vi "Configure Input Wavelength.vi"(0 "VISA resource name":refnum<visa-resource-name>, 1 "Wavelength Unit (0:NM)":u16(ring) items=["NM", "M"], 5 "Platform Slot Number (10)":i16=10 min=-1 max=255, 7 "Wavelength (0:MINimum)":i32(ring) items=["MINimum", "MAXimum", "DEFault", "User Defined Value"], 9 "User Defined Wavelength Value (1310)":dbl=1310.0, 11 "error in (no error)":errorcluster) -> (4 "VISA resource name out":refnum<visa-resource-name>, 15 "error out":errorcluster)   [LabVIEW 2018, in "LTB-1.lvlib" / "3150.lvlib"]
doc: "Configures the specific Input wavelength in meters or nanometers"
uses:
  3150.lvlib
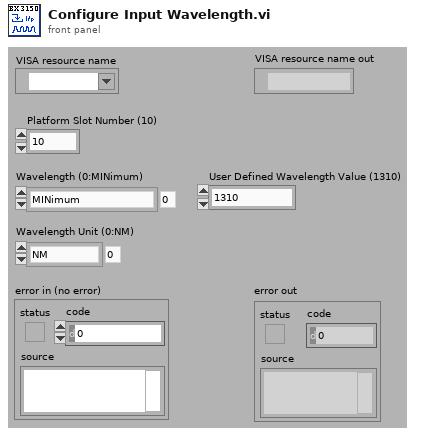
[diagram p1: front panel]
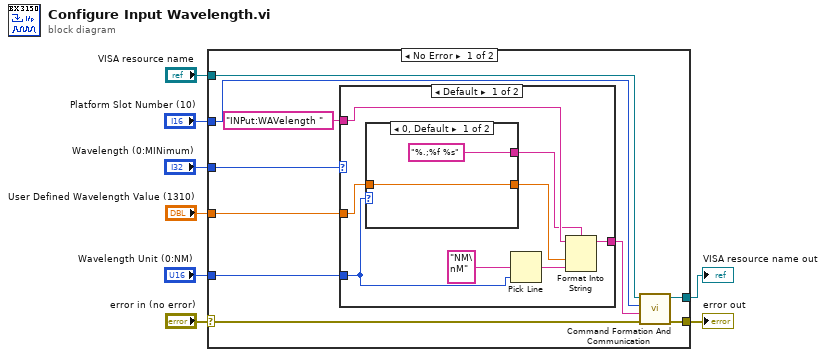
[diagram p0: block diagram]
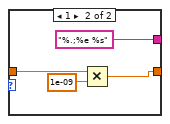
[diagram p2: hidden frame]
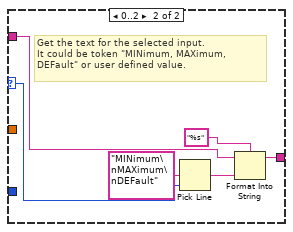
[diagram p3: hidden frame]
diagram:
  n1 = case shown="No Error" "error in (no error)" {
    selector: "error in (no error)" -> [w13 w40]
    tunnel: "VISA resource name" -> [w15 w39]
    tunnel: [w11 w40] -> w6
    tunnel: "Wavelength (0:MINimum)" -> [w10 _]
    tunnel: "Wavelength Unit (0:NM)" -> [w18 _]
    tunnel: "Platform Slot Number (10)" -> [w14 _]
    tunnel: [w12 w39] -> w2
    tunnel: "User Defined Wavelength Value (1310)" -> [w9 _]
    frame No Error {
      n2 = case shown="Default" w10 {
        selector: w10 -> [_ w34]
        tunnel: w18 -> [w20 _]
        tunnel: "INPut:WAVelength " ("Command") -> [w24 w35]
        tunnel: [w23 w33] -> w16
        tunnel: w9 -> [w22 _]
        frame Default {
          n3 = case shown="0, Default" w20 {
            tunnel: w22 -> [w28 w32]
            tunnel: [w28 w30] -> w21
            tunnel: ["%.;%f %s" ("format string") "%.;%e %s" ("format string")] -> w19
            frame 0, Default {
            }
            frame 1 {
              n4 = Multiply(x=w32, y=1e-09) -> (x*y=w30:dbl)
            }
          }
          n5 = Pick Line(multi-line string="NM\nM", line index=w20) -> (output string=w25:string)  [unwired: 1 out]
          n6 = Format Into String(format string=w19, initial string=w24, w21, w25) -> (resulting string=w23:string)  [unwired: 1 in, 1 out]
        }
        frame 0..2 {
          # "Get the text for the selected input.\nIt could be token \"MINimum, MAXimum,\nDEFault\" or user defined value."
          n7 = Pick Line(multi-line string="MINimum\nMAXimum\nDEFault", line index=w34) -> (output string=w36:string)  [unwired: 1 out]
          n8 = Format Into String(format string="%s", initial string=w35, w36) -> (resulting string=w33:string)  [unwired: 1 in, 1 out]
        }
      }
      n9 = call "Command Formation And Communication.vi"("error in (no error)"=w13, "Command"=w16, "Platform Slot Number"=w14, "VISA resource name"=w15) -> ("error out"=w11:errorcluster, "VISA resource name out"=w12:refnum<visa-resource-name>)  [unwired: 6 out]
    }
    frame Error {
    }
  }
  "VISA resource name out" <- w2
  "error out" <- w6
